vi "Sub Initialize.vi"(8 "error in (no error)":errorcluster, 11 "Instrument Recorder in":refnum<class "Instrument Recorder.lvclass">) -> (0 "error out":errorcluster, 2 "Initialize Result":refnum<class "Acquired Result.lvclass">, 3 "Instrument Recorder out":refnum<class "Instrument Recorder.lvclass">)   [LabVIEW 2015, in "Instrument Recorder.lvclass"]
uses:
  Instrument Recorder.lvclass
  Results/Acquired Result/Acquired Result.lvclass
  Instrument Recorder.lvclass/Instrument Recorder.ctl
  Read Instrument driver.vi
  Write Instrument driver.vi
  NHMFL_Core/Libraries/Instruments/Instrument Driver/Instrument Driver.lvclass
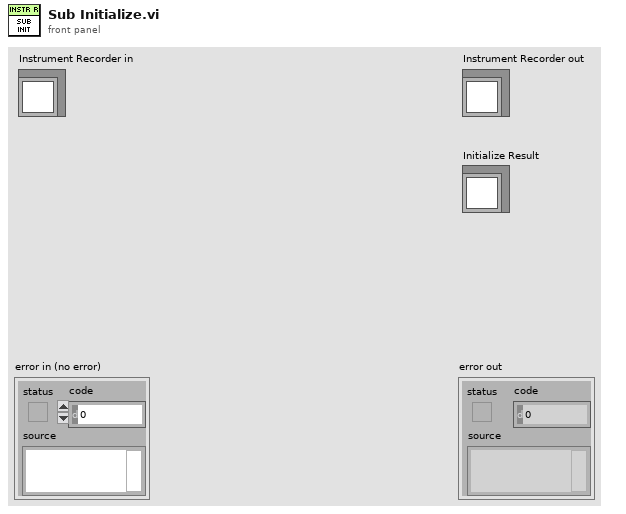
[diagram p1: front panel]
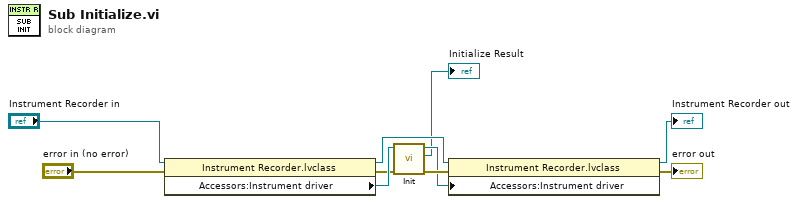
[diagram p0: block diagram]
diagram:
  n1 = property class="Instrument Recorder.lvclass"(reference="Instrument Recorder in", error in="error in (no error)") -> (reference out=w8:refnum<class "Instrument Recorder.lvclass">, error out=w7:errorcluster, "Accessors:Instrument driver"=w9:refnum<class "Instrument Driver.lvclass">)
  n2 = call-dynamic "Init.vi"("error in (no error)"=w7, "Instrument Driver in"=w9) -> ("error out"=w5:errorcluster, "Init Result"=→"Initialize Result":refnum<class "Acquired Result.lvclass">, "Instrument Driver out"=w4:refnum<class "Instrument Driver.lvclass">)  [unwired: 7 in]
  n3 = property class="Instrument Recorder.lvclass"(reference=w8, error in=w5, "Accessors:Instrument driver"=w4) -> (reference out=→"Instrument Recorder out":refnum<class "Instrument Recorder.lvclass">, error out=→"error out":errorcluster)
